vi "Spark Statistics to Acnet Writer.vi"() -> ()   [LabVIEW 2012]
uses:
  DWP Scope VIs/201 MHz Global Cavity Variables.vi
panel:
  in  "Device 2":string="E:C2PRSK"
  out "Probe V of Last Spark":dbl
  out "Loops":i32=12
  out "Local Stop":bool
  out "Is Playing?":bool
  in  "Test the sound":bool
  in  "Sound File Path":path=path "C:/LabVIEW for MTA/DaveP/LabVIEW Development/LabVIEW 2012 versions/Dave's Test VIs/Sound Files/HPRF Single Spark Slowest.wav"
  in  "Device":string="E:C2SPTM"
  out "Recent Spark Intervals":i32[](array[numeric])
  in  "stop":bool
  out "Pulses since Last Spark":i32
  # "Spark Statistics to Acnet Writer.vi\n27 Mar 2013\nby D. Peterson"
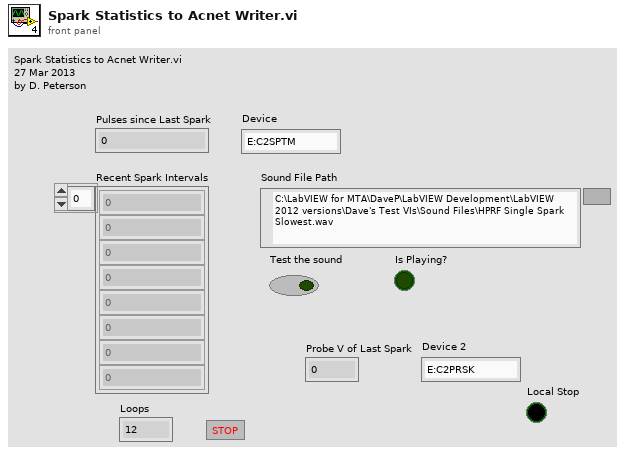
[diagram p1: front panel]
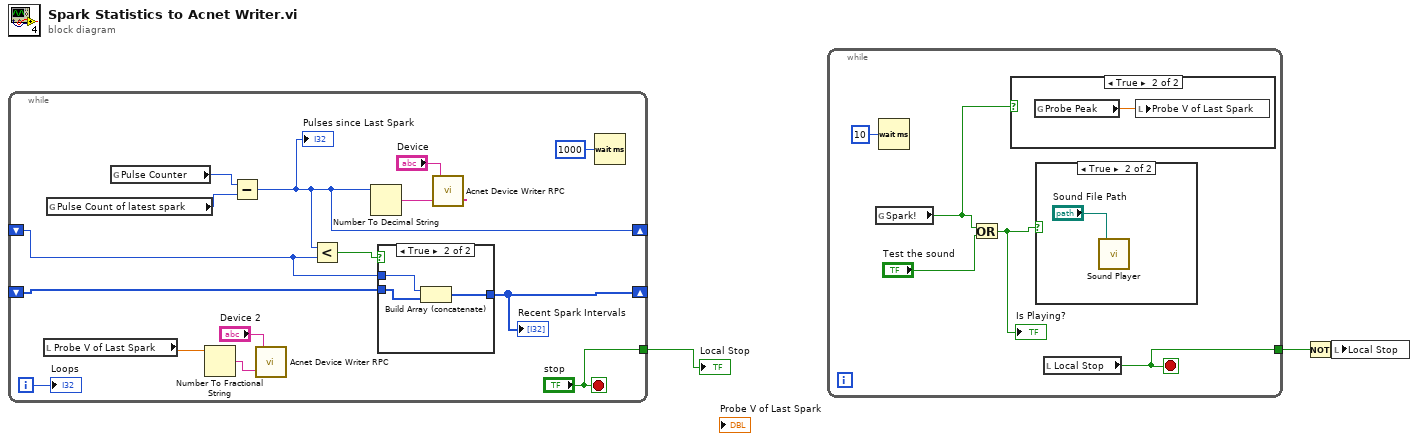
[diagram p0: block diagram]
diagram:
  n1 = while {
    shift-right: [w9] -> _
    shift-left: _ -> [w12]
    shift-right: [w14] -> _
    shift-left: _ -> [w13]
    tunnel: ["stop"] -> w1
    i -> [w7]
    stop <- "stop" stop-if-true
    n2 = local read "Probe V of Last Spark"() -> (w4:dbl)
    n3 = global read "201 MHz Global Cavity Variables.vi" "Pulse Count of latest spark"() -> (w17:i32)
    n4 = global read "201 MHz Global Cavity Variables.vi" "Pulse Counter"() -> (w18:i32)
    n5 = Number To Fractional String(number=w4) -> (F-format string=w5:string)  [unwired: 3 in]
    n6 = Subtract(x=w18, y=w17) -> (x-y=w9:i32)
    "Pulses since Last Spark" <- w9
    n7 = call "Acnet Device Writer RPC.vi"("Value"=w5, "Device"="Device 2") -> ()  [unwired: 1 in]
    n8 = Less?(x=w9, y=w12) -> (x < y?=w15:bool)
    n9 = Number To Decimal String(number=w9) -> (decimal integer string=w10:string)  [unwired: 1 in]
    n10 = case shown="True" w15 {
      tunnel: w12 -> [_ w21]
      tunnel: [w19 w22] -> w14
      tunnel: w13 -> [w19 w20]
      frame False {
      }
      frame True {
        n11 = Build Array (concatenate)(w21, w20) -> (w22:i32[])
      }
    }
    "Recent Spark Intervals" <- w14
    n12 = call "Acnet Device Writer RPC.vi"("Value"=w10, "Device"="Device") -> ()  [unwired: 1 in]
    n13 = Wait (ms)(milliseconds to wait=u32 1000) -> ()  [unwired: 1 out]
    "Loops" <- w7
  }
  "Local Stop" <- w1
  n14 = while {
    tunnel: [w25] -> w3
    stop <- w25 stop-if-true
    n15 = global read "201 MHz Global Cavity Variables.vi" "Spark!"() -> (w23:bool)
    n16 = Wait (ms)(milliseconds to wait=u32 10) -> ()  [unwired: 1 out]
    n17 = Or(x=w23, y="Test the sound") -> (x .or. y?=w24:bool)
    "Is Playing?" <- w24
    n18 = case shown="True" w23 {
      frame False {
      }
      frame True {
        n19 = global read "201 MHz Global Cavity Variables.vi" "Probe Peak"() -> (w28:dbl)
        n20 = local write "Probe V of Last Spark"(w28) -> ()
      }
    }
    n21 = case shown="True" w24 {
      frame False {
      }
      frame True {
        n22 = call "Sound Player.vi"("Sound File Path"="Sound File Path") -> ()  [unwired: 4 in, 1 out]
      }
    }
    n23 = local read "Local Stop"() -> (w25:bool)
  }
  n24 = Not(x=w3) -> (.not. x?=w2:bool)
  n25 = local write "Local Stop"(w2) -> ()
